vi "Example_OE1201 Control.vi"() -> ()   [LabVIEW 2011]
panel:
  in  "Sample count":u32
  out "Gain Overlaod":bool
  in  "Remote Mode":u16(ring) items=["USB", "RS232"]
  out "Freq":dbl
  out "xita":dbl
  out "R":dbl
  out "Input Overlaod":bool
  out "PLL Lock":bool
  out "Error":string
  out "Serial Versions":string
  in  "Table":T1(tab) caption="选项卡控件"
  in  "OE1201_Configure Input Filter":T2 {"Input Notch Filter" items=["None", "50Hz", "100Hz", "Both"]; "Input Coupling" items=["AC", "DC"]; "Input Shield Grounding" items=["Float", "Ground"]; "Input Source" items=["A", "B", "I-1M", "I-100M"]}
  in  "OE1201_Configure Ref Phase":T3={"Internal Frequency(Hz)"=1000.0, "External Ref Trigger"=0, "Reference Source"=0, "Phase  (degree)"=0.0} {"Phase  (degree)" format="%#.2g"; "Reference Source" items=["External", "Internal"]; "External Ref Trigger" items=["TTL Rising Edge", "Sine Zero Crossing"]; "Internal Frequency(Hz)" min=0.001 max=120000.0 format="%#_10g"}
  in  "OE1201_Configure Sens and Filter":T4={"Dynamic Reserve"=1, "Sensitivity "=24, "Time Constant "=9, "Low Pass Filter Slope "=1, "Enable Sync Filter "=0} {"Enable Sync Filter" items=["OFF", "ON"]; "Low Pass Filter Slope" items=["6 dB/oct", "12 dB/oct", "18 db/oct", "24 dB/oct"]; "Time Constant" items=["10 us", "30 us", "100 us", "300 us", "1 ms", "3 ms", "10 ms", "30 ms", "100 ms", "300 ms", "1 s", "3 s", "10 s", "30 s", "100 s", "300 s", "1 ks", "3 ks"]; "Sensitivity" items=["2 nV/fA", "5 nV/fA", "10 nV/fA", "20 nV/fA", "50 nV/fA", "100 nV/fA", "200 nV/fA", "500 nV/fA", "1 uV/pA", "2 uV/pA", "5 uV/pA", "10 uV/pA", "20 uV/pA", "50 uV/pA", "100 uV/pA", "200 uV/pA", "500 uV/pA", "1 mV/nA", "2 mV/nA", "5 mV/nA", "10 mV/nA", "20 mV/nA", "50 mV/nA", "100 mV/nA", "200 mV/nA", "500 mV/nA", "1 V/uA"]; "Dynamic Reserve" items=["High Reserve", "Normal", "Low Noise"]}
  in  "OE1201_Configure Channel Out":T5={"CH 1"=0, "CH 2"=0, "CH2 Offset(%)"=0.0, "CH1 Offset(%)"=0.0, "CH2 Expand"=1, "CH1 Expand"=1} {"CH1 Expand" min=1 max=256; "CH2 Expand" min=1 max=256; "CH1 Offset(%)" min=-100.0 max=100.0 format="%#.2g"; "CH2 Offset(%)" min=-100.0 max=100.0 format="%#.2g"; "CH 2" items=["R"=3, "X"=1, "Y"=2, "θ"=4]; "CH 1" items=["R"=3, "X"=1, "Y"=2, "θ"=4]}
  in  "OE1201_Configure Sine Out":cluster{"Sine Output Amplitude (V)":dbl}={"Sine Output Amplitude (V)"=0.1} {"Sine Output Amplitude (V)" min=0.1 max=1.0 format="%.3f"}
  in  "OE1201_Configure Harmonic":cluster{"Harmonic":u16}={"Harmonic"=1} {"Harmonic" min=1 max=32767}
  in  "Sample Rate":dbl=0.1 min=0.1 max=100.0
  in  "Save Button":bool
  in  "file path":path
  out "Status":string
  in  "Connect":bool
  in  "VISA resource name":refnum<visa-resource-name>
  in  "Baud Rate (921600)":u32=921600
  # "Tel          :   +86-020-84133345\nWebsite  :   www.ssi-instrument.com\nE-mail     :   support@si-instrument.com"
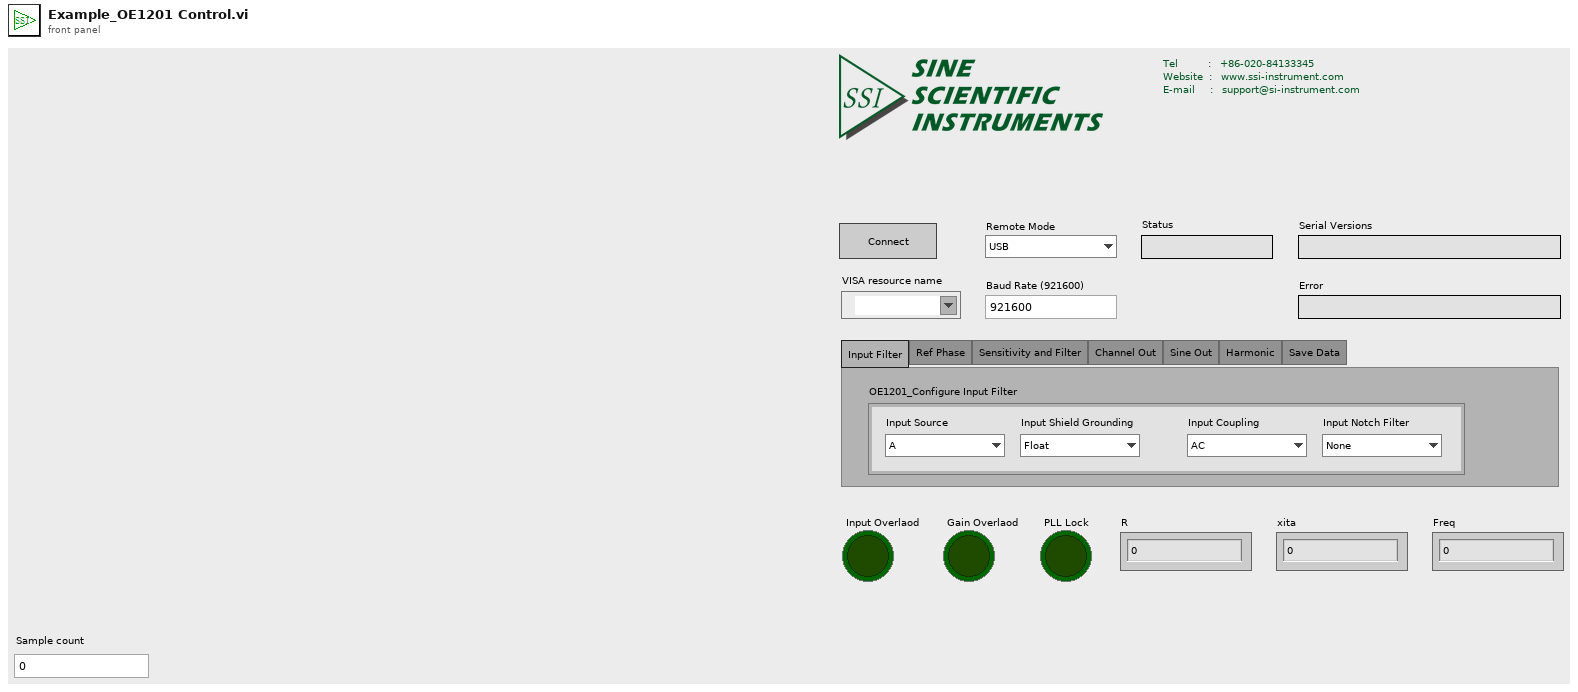
[diagram p1: front panel]
types:
  T1 = enum32{"Input Filter", "Ref Phase", "Sensitivity and Filter", "Channel Out", "Sine Out", "Harmonic", "Save Data"}
  T2 = cluster{"Input Source":u16, "Input Shield Grounding ":u16, "Input Coupling ":u16, "Input Notch Filter ":u16}
  T3 = cluster{"Internal Frequency(Hz)":dbl, "External Ref Trigger":u16, "Reference Source":u16, "Phase  (degree)":dbl}
  T4 = cluster{"Dynamic Reserve":u16, "Sensitivity ":u16, "Time Constant ":u8, "Low Pass Filter Slope ":u8, "Enable Sync Filter ":u16}
  T5 = cluster{"CH 1":i8, "CH 2":i8, "CH2 Offset(%)":dbl, "CH1 Offset(%)":dbl, "CH2 Expand":u16, "CH1 Expand":u16}
  T6 = enum16{"OE1022", "OE1022D", "OE1201", "OE2031&OE2041", "OE1311&OE1351"}
  T7 = cluster{"Input Overlaod":bool, "Gain Overlaod":bool, "PLL Lock(1: External Lock)":bool}
  T8 = cluster{"R":dbl, "X":dbl, "Y":dbl, "θ":dbl, "Freq":dbl}
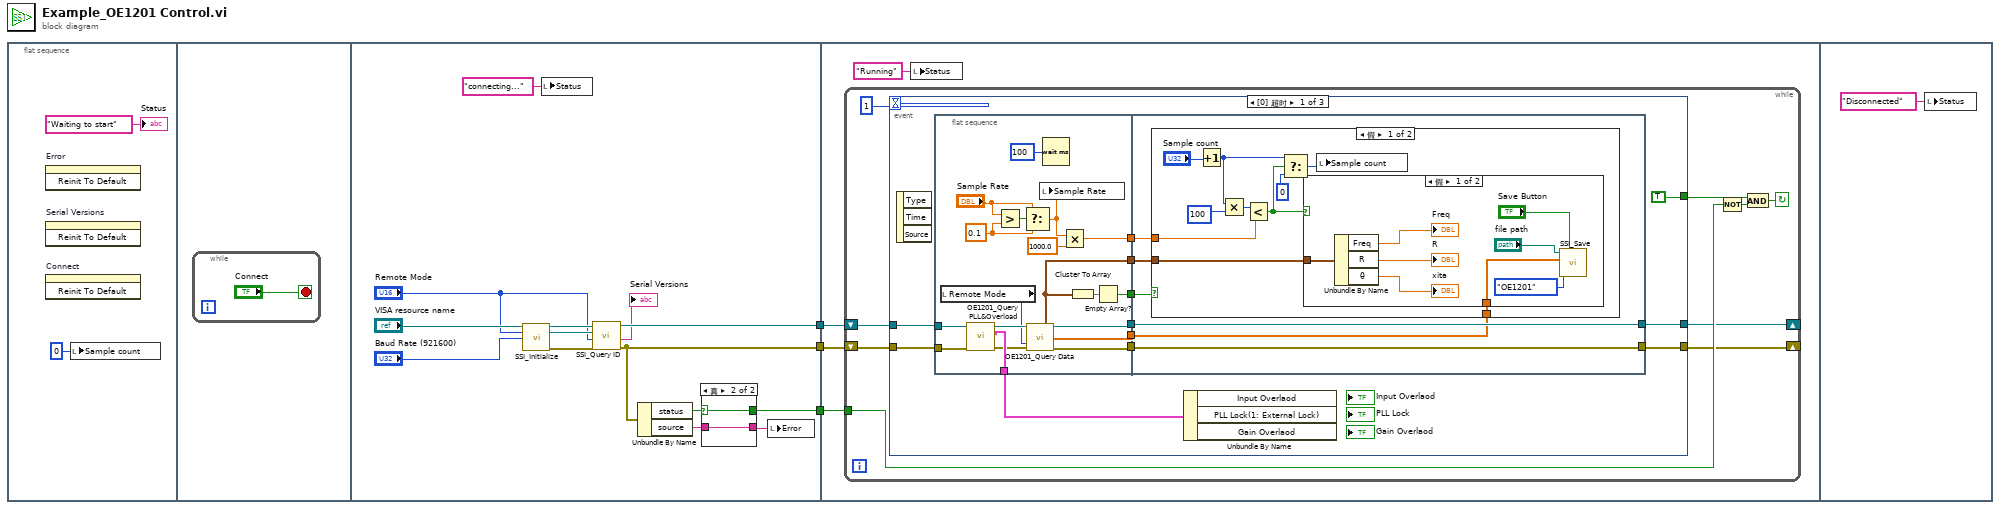
[diagram p0: block diagram]
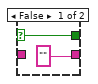
[diagram p2: hidden frame]
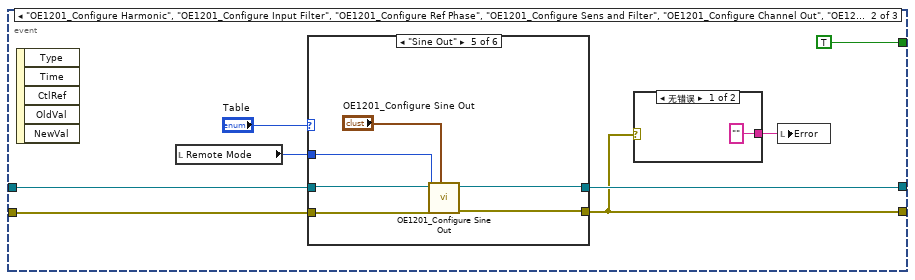
[diagram p5: hidden frame]
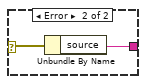
[diagram p6: hidden frame]
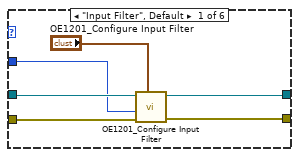
[diagram p7: hidden frame]
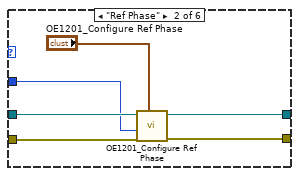
[diagram p8: hidden frame]
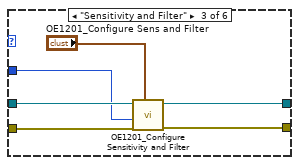
[diagram p9: hidden frame]
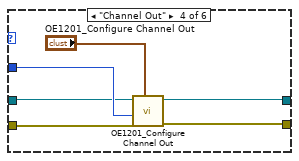
[diagram p10: hidden frame]
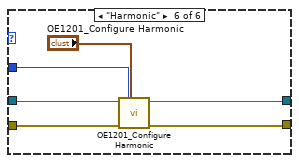
[diagram p11: hidden frame]
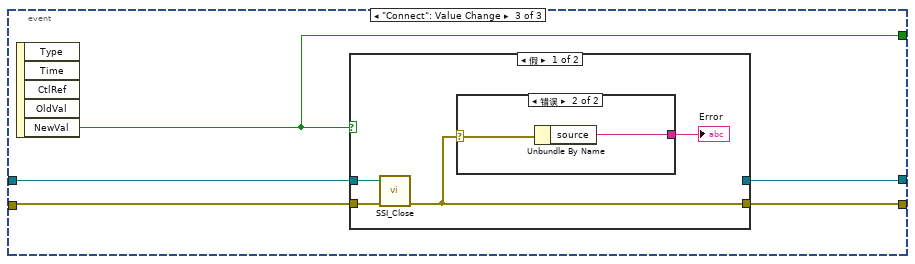
[diagram p12: hidden frame]
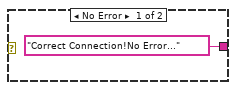
[diagram p13: hidden frame]
diagram:
  n1 = flat-sequence {
    tunnel: [w14] -> w3
    tunnel: [w11] -> w2
    tunnel: [w9] -> w1
    tunnel: w3 -> [w27]
    tunnel: w2 -> [w26]
    tunnel: w1 -> [w25]
    frame #0 {
      n2 = invoke on="Error" class="Str" method="Reinit To Default"() -> ()  [unwired: 3 in, 3 out]
      n3 = invoke on="Serial Versions" class="Str" method="Reinit To Default"() -> ()  [unwired: 3 in, 3 out]
      n4 = invoke on="Connect" class="Bool (严格)" method="Reinit To Default"() -> ()  [unwired: 3 in, 3 out]
      n5 = local write "Sample count"(u32 0 ("Sample count")) -> ()
      "Status" <- "Waiting to start" ("status")
    }
    frame #1 {
      n6 = while {
        stop <- "Connect" stop-if-true
      }
    }
    frame #2 {
      n7 = call "SSI_Initialize.vi"("VISA resource name"="VISA resource name", "Remote Mode"="Remote Mode", "baud rate (921600)"="Baud Rate (921600)") -> ("VISA resource name out"=w18:refnum<visa-resource-name>, "connection ID(Ethernet)"=w17:refnum<k5>, "error out"=w16:errorcluster)  [unwired: 10 in]
      n8 = local write "Status"("connecting..." ("status")) -> ()
      n9 = call "SSI_Query ID.vi"("Error in (no error)"=w16, "Remote Mode"="Remote Mode", "Connection ID in"=w17, "VISA resource name"=w18) -> ("Error out"=w11:errorcluster, "Read Buffer"=→"Serial Versions":string, "VISA resource  out"=w14:refnum<visa-resource-name>)  [unwired: 4 in, 1 out]
      n10 = Unbundle By Name(w11) -> ("status"=w10:bool, "source"=w8:string)
      n11 = case shown="真" w10 {
        selector: w10 -> [w22 w24]
        tunnel: [w22 w24] -> w9
        tunnel: ["" w23] -> w7
        tunnel: w8 -> [_ w23]
        frame False {
        }
        frame True {
        }
      }
      n12 = local write "Error"(w7) -> ()
    }
    frame #3 {
      n13 = while {
        tunnel: w25 -> [w33]
        shift-right: [w30] -> _
        shift-left: w27 -> [w31]
        shift-right: [w29] -> _
        shift-left: w26 -> [w32]
        stop <- w34 continue-if-true
        n14 = event shown="[0] 超时" {
          selector: _ -> [_ _ _]
          dyn-events: _ -> [_ _ _]
          timeout: 1 -> [_ _ _]
          tunnel: [TRUE ("Stop") TRUE ("Stop") w140] -> w35
          tunnel: [w44 w95 w142] -> w29
          tunnel: [w45 w97 w141] -> w30
          tunnel: w31 -> [w46 w99 w144]
          tunnel: w32 -> [w47 w98 w143]
          event Timeout {
            n15 = event-data() -> ()  [unwired: 1 in, 3 out]
            n16 = flat-sequence {
              tunnel: [w55] -> w43
              tunnel: [w56] -> w42
              tunnel: [w63] -> w41
              tunnel: [w62] -> w40
              tunnel: [w51] -> w39
              tunnel: [w52] -> w38
              tunnel: [w54] -> w48
              tunnel: w47 -> [w58]
              tunnel: w46 -> [w59]
              tunnel: w43 -> [w73]
              tunnel: w42 -> [w74]
              tunnel: [w74] -> w45
              tunnel: [w73] -> w44
              tunnel: w41 -> [w70]
              tunnel: w40 -> [w69]
              tunnel: w39 -> [w71]
              tunnel: w38 -> [w72]
              frame #0 {
                w66 = 0.1 ("y")
                n17 = local read "Remote Mode"() -> (w50:u16)
                n18 = call "OE1201_Query PLL&Overload.vi"("Error in (no error)"=w58, "VISA resource name"=w59) -> ("Error out"=w53:errorcluster, "OE1201_Query PLL&Overload"=w54:T7, "VISA resource  out"=w57:refnum<visa-resource-name>)  [unwired: 6 in, 1 out]
                n19 = Greater?(x="Sample Rate", y=w66) -> (0:w65:bool)
                n20 = Select(t="Sample Rate", s=w65, f=w66) -> (s? t:f=w64:dbl)
                n21 = call "OE1201_Query Data.vi"("VISA resource name"=w57, "Remote Mode"=w50, "Error in (no error)"=w53) -> ("VISA resource  out"=w56:refnum<visa-resource-name>, "Parameter Values"=w51:T8, "Data Array"=w52:dbl[], "Error out"=w55:errorcluster)  [unwired: 8 in, 1 out]
                n22 = local write "Sample Rate"(w64) -> ()
                n23 = Wait (ms)(milliseconds to wait=u32 100 ("等待时间（毫秒）")) -> ()  [unwired: 1 out]
                n24 = Multiply(x=w64, y=1000.0) -> (x*y=w62:dbl)
                n25 = Cluster To Array(cluster=w51) -> (array=w68:dbl[])
                n26 = Empty Array?(array=w68) -> (empty?=w63:bool)
              }
              frame #1 {
                n27 = case shown="假" w70 {
                  tunnel: w72 -> [w84 _]
                  tunnel: w71 -> [w83 _]
                  tunnel: w69 -> [w80 _]
                  frame False {
                    n28 = Increment(x="Sample count") -> (x+1=w76:u32)
                    n29 = Multiply(x=w76, y=u32 100) -> (x*y=w81:u32)
                    n30 = Less?(x=w81, y=w80) -> (x < y?=w78:bool)
                    n31 = Select(t=w76, s=w78, f=0) -> (s? t:f=w77:u32)
                    n32 = case shown="假" w78 {
                      tunnel: w83 -> [w92 _]
                      tunnel: w84 -> [w91 _]
                      frame False {
                        n33 = Unbundle By Name(w92) -> ("Freq"=→"Freq":dbl, "R"=→"R":dbl, "θ"=→"xita":dbl)
                        n34 = call "SSI_Save.vi"("file path (dialog if empty)"="file path", "1D data"=w91, "Instrument Mode"=T6."OE1201", "Save Button"="Save Button") -> ()  [unwired: 7 in]
                      }
                      frame True {
                      }
                    }
                    n35 = local write "Sample count"(w77) -> ()
                  }
                  frame True {
                  }
                }
              }
            }
            n36 = Unbundle By Name(w48) -> ()  [unwired: 3 out]
          }
          event "OE1201_Configure Harmonic", "OE1201_Configure Input Filter", "OE1201_Configure Ref Phase", "OE1201_Configure Sens and Filter", "OE1201_Configure Channel Out", "OE1201_Configure Sine Out": Value Change {
            n37 = event-data() -> ()  [unwired: 1 in, 5 out]
            n38 = local read "Remote Mode"() -> (w93:u16)
            n39 = case shown="\"Sine Out\"" "Table" {
              tunnel: w99 -> [w108 w115 w121 w125 w130 w137]
              tunnel: w98 -> [w109 w114 w120 w127 w133 w139]
              tunnel: [w106 w113 w118 w123 w131 w136] -> w97
              tunnel: [w107 w112 w119 w124 w132 w135] -> w95
              tunnel: w93 -> [w105 w111 w117 w126 w129 w138]
              frame "Input Filter", Default {
                n40 = call "OE1201_Configure Input Filter.vi"("OE1201_Configure Input Filter"="OE1201_Configure Input Filter", "Error in (no error)"=w109, "Remote Mode"=w105, "VISA resource name"=w108) -> ("Error out"=w107:errorcluster, "VISA resource  out"=w106:refnum<visa-resource-name>)  [unwired: 5 in, 1 out]
              }
              frame "Ref Phase" {
                n41 = call "OE1201_Configure Ref Phase.vi"("OE1201_Configure Ref Phase"="OE1201_Configure Ref Phase", "Error in (no error)"=w114, "Remote Mode"=w111, "VISA resource name"=w115) -> ("Error out"=w112:errorcluster, "VISA resource  out"=w113:refnum<visa-resource-name>)  [unwired: 5 in, 1 out]
              }
              frame "Sensitivity and Filter" {
                n42 = call "OE1201_Configure Sensitivity and Filter.vi"("OE1201_Configure Sens and Filter"="OE1201_Configure Sens and Filter", "Error in (no error)"=w120, "Remote Mode"=w117, "VISA resource name"=w121) -> ("Error out"=w119:errorcluster, "VISA resource  out"=w118:refnum<visa-resource-name>)  [unwired: 5 in, 1 out]
              }
              frame "Channel Out" {
                n43 = call "OE1201_Configure Channel Out.vi"("OE1201_Configure Channel Out"="OE1201_Configure Channel Out", "Error in (no error)"=w127, "Remote Mode"=w126, "VISA resource name"=w125) -> ("Error out"=w124:errorcluster, "VISA resource  out"=w123:refnum<visa-resource-name>)  [unwired: 5 in, 1 out]
              }
              frame "Sine Out" {
                n44 = call "OE1201_Configure Sine Out.vi"("OE1201_Configure Sine Out"="OE1201_Configure Sine Out", "Error in (no error)"=w133, "Remote Mode"=w129, "VISA resource name"=w130) -> ("Error out"=w132:errorcluster, "VISA resource  out"=w131:refnum<visa-resource-name>)  [unwired: 5 in, 1 out]
              }
              frame "Harmonic" {
                n45 = call "OE1201_Configure Harmonic.vi"("OE1201_Configure Harmonic"="OE1201_Configure Harmonic", "Error in (no error)"=w139, "Remote Mode"=w138, "VISA resource name"=w137) -> ("Error out"=w135:errorcluster, "VISA resource  out"=w136:refnum<visa-resource-name>)  [unwired: 5 in, 1 out]
              }
            }
            n46 = case shown="无错误" w95 {
              selector: w95 -> [_ w103]
              tunnel: ["" ("source") w102] -> w94
              frame No Error {
              }
              frame Error {
                n47 = Unbundle By Name(w103) -> ("source"=w102:string)
              }
            }
            n48 = local write "Error"(w94) -> ()
          }
          event "Connect": Value Change {
            n49 = event-data() -> ("NewVal"=w140:bool)  [unwired: 1 in, 4 out]
            n50 = case shown="假" w140 {
              tunnel: w144 -> [w148 w153]
              tunnel: w143 -> [w147 w152]
              tunnel: [w146 w152] -> w142
              tunnel: [_ w153] -> w141
              frame False {
                n51 = call "SSI_Close.vi"("Error in (no error)"=w147, "VISA resource name"=w148) -> ("Error out"=w146:errorcluster)  [unwired: 5 in]
                n52 = case shown="错误" w146 {
                  selector: w146 -> [_ w151]
                  tunnel: ["Correct Connection!No Error..." ("source") w150] -> w145
                  frame No Error {
                  }
                  frame Error {
                    n53 = Unbundle By Name(w151) -> ("source"=w150:string)
                  }
                }
                "Error" <- w145
              }
              frame True {
              }
            }
          }
        }
        n54 = Not(x=w33) -> (.not. x?=w36:bool)
        n55 = And(x=w35, y=w36) -> (x .and. y?=w34:bool)
      }
      n56 = local write "Status"("Running" ("status")) -> ()
    }
    frame #4 {
      n57 = local write "Status"("Disconnected" ("status")) -> ()
    }
  }
